vi "Stop Core.vi"(10 "final error code":i32, 11 "Client UI in":refnum<class "Client UI.lvclass">) -> (3 "Client UI out":refnum<class "Client UI.lvclass">)   [LabVIEW 2015, in "Client UI.lvlib" / "Client UI.lvclass"]
uses:
  Client UI.lvclass
  <userlib>/Common Components/Msmt UI/Measurement UI.lvclass
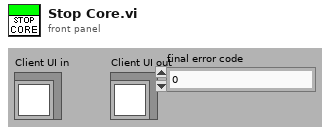
[diagram p1: front panel]
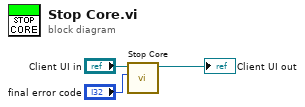
[diagram p0: block diagram]
diagram:
  n1 = call-parent "Stop Core.vi"("final error code"="final error code", "Operator UI Actor in"="Client UI in") -> ("Operator UI Actor out"=→"Client UI out":refnum<class "Client UI.lvclass">)  [unwired: 9 in]
